vi "Search 1 D Array Index Element.vi"() -> ()   [LabVIEW 2015]
panel:
  in  "Tab Control":enum32{"Page 1", "Page 2"}(tab)
  out "index of element":i32
  in  "element":dbl
  out "Array":dbl[](array[numeric])
  # "Search 1 D Array Index Element"
  # "Pardeep Kumar"
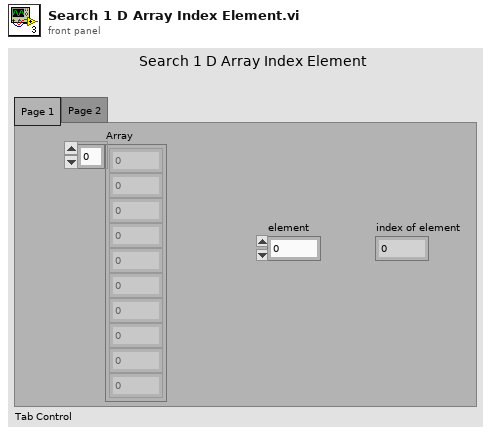
[diagram p1: front panel]
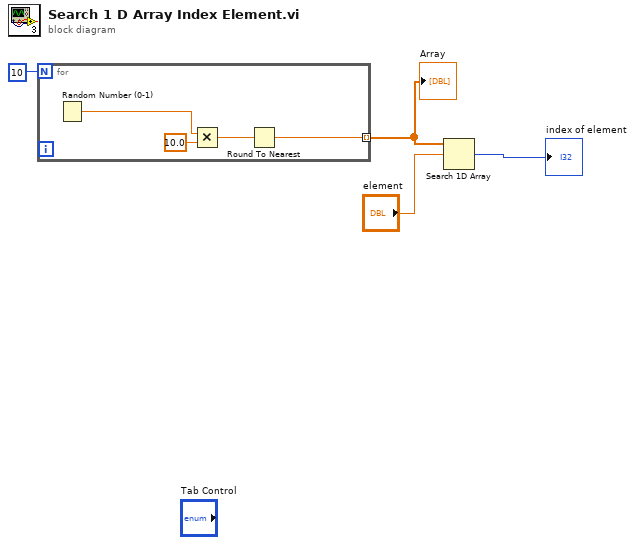
[diagram p0: block diagram]
diagram:
  n1 = for {
    N: 10 -> [_]
    tunnel: [w5] -> w4 mode=indexing
    n2 = Random Number (0-1)() -> (number: 0 to 1=w8:dbl)
    n3 = Multiply(x=w8, y=10.0) -> (x*y=w6:dbl)
    n4 = Round To Nearest(number=w6) -> (nearest integer value=w5:dbl)
  }
  "Array" <- w4
  n5 = Search 1D Array(1D array=w4, element="element") -> (index of element=→"index of element":i32)  [unwired: 1 in]
